vi "Build UEGO Section.vi"(6 "Cancelled?":bool, 7 "FPGA Item Name":string, 8 "error in (no error)":errorcluster, 9 "Card Position in":T1 {"Slot #" max=15}, 10 "Name in":string, 11 "Node Ptr in":u64) -> (0 "error out":errorcluster)   [LabVIEW 2014, in "SLSC configuration System Explorer.lvlib"]
uses:
  SLSC configuration System Explorer.lvlib
  Type Defs/Card Position.ctl
  Shared/SPI Utility/Slot #.ctl
  Shared/Constants.vi
  <vilib>/NI Veristand/Custom Device API/Set Item Property (U32).vi
  <vilib>/NI Veristand/Custom Device API/Set Item Property (String).vi
  <vilib>/NI Veristand/Custom Device API/Custom Device API.lvlib
  Shared/SLSC configuration Shared.lvlib
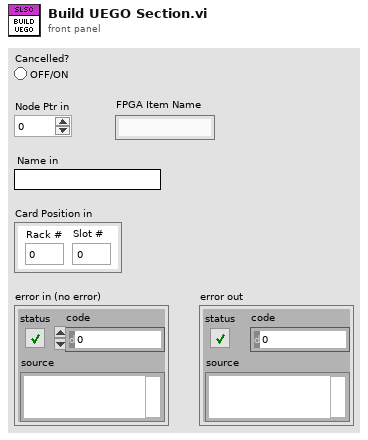
[diagram p1: front panel]
types:
  T1 = typedef "SLSC configuration Shared.lvlib/Card Position.ctl" = cluster{"Rack #":u8, "Slot #":T2}
  T2 = typedef "SLSC configuration Shared.lvlib/Slot #.ctl" = u8
  T3 = typedef "Custom Device API.lvlib/Custom Device Item Ref.ctl" = u64
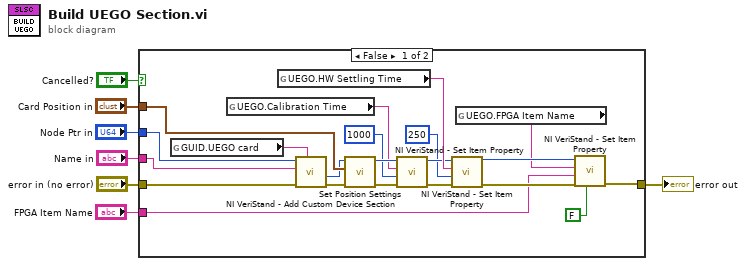
[diagram p0: block diagram]
diagram:
  n1 = case shown="False" "Cancelled?" {
    tunnel: "error in (no error)" -> [w27 w29]
    tunnel: "Name in" -> [w26 _]
    tunnel: "Node Ptr in" -> [w25 _]
    tunnel: "Card Position in" -> [w23 _]
    tunnel: [w11 w29] -> w6
    tunnel: "FPGA Item Name" -> [w8 _]
    frame False {
      n2 = global read "Constants.vi" "GUID.UEGO card"() -> (w28:string)
      n3 = global read "Constants.vi" "UEGO.Calibration Time"() -> (w19:string)
      n4 = global read "Constants.vi" "UEGO.HW Settling Time"() -> (w18:string)
      n5 = call <vilib>:"NI VeriStand - Add Custom Device Section.vi"("GUID (Default Section)"=w28, "error in (no error)"=w27, "Section Name"=w26, "Parent Ref in"=w25) -> ("error out"=w24:errorcluster, "Section Ptr"=w22:T3)  [unwired: 4 in, 2 out]
      n6 = call "Set Position Settings.vi"("error in (no error)"=w24, "Card Position"=w23, "Item Ref in"=w22) -> ("error out"=w21:errorcluster, "Item Ref out"=w20:T3)  [unwired: 7 in]
      n7 = call-poly <vilib>:"NI VeriStand - Set Item Property.vi"("error in (no error)"=w21, "Value"=u32 1000, "Property Name"=w19, "Item Ref in"=w20) -> ("error out"=w16:errorcluster, "Item Ref out"=w17:T3)  [unwired: 5 in, 1 out]
      n8 = call-poly <vilib>:"NI VeriStand - Set Item Property.vi"("error in (no error)"=w16, "Value"=u32 250, "Property Name"=w18, "Item Ref in"=w17) -> ("error out"=w13:errorcluster, "Item Ref out"=w12:T3)  [unwired: 5 in, 1 out]
      n9 = global read "Constants.vi" "UEGO.FPGA Item Name"() -> (w10:string)
      n10 = call-poly <vilib>:"NI VeriStand - Set Item Property.vi"("Binary String (T)"=FALSE, "error in (no error)"=w13, "Value"=w8, "Property Name"=w10, "Item Ref in"=w12) -> ("error out"=w11:errorcluster)  [unwired: 4 in, 2 out]
    }
    frame True {
    }
  }
  "error out" <- w6
